vi "Read SMO Address.vi"(8 "error in (no error)":errorcluster, 11 "Instrument in":refnum<class "Instrument.lvclass">) -> (0 "error out":errorcluster, 2 "Address":string, 3 "Instrument out":refnum<class "Instrument.lvclass">)   [LabVIEW 2019, in "Instrument.lvclass"]
uses:
  Instrument.lvclass
  Instrument.lvclass/Instrument.ctl
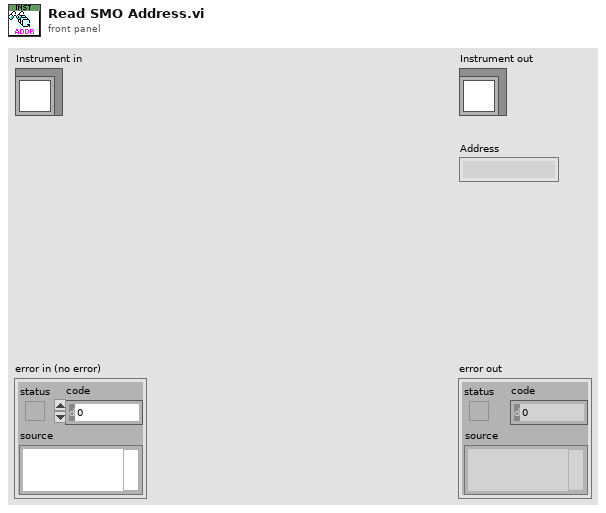
[diagram p1: front panel]
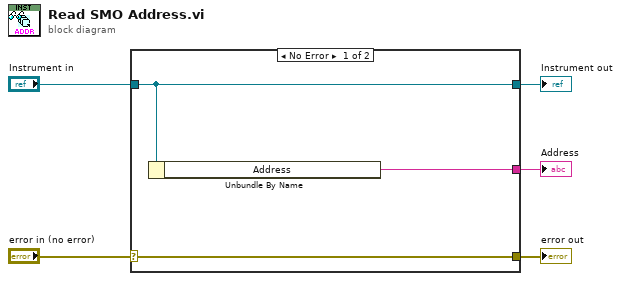
[diagram p0: block diagram]
diagram:
  n1 = case shown="No Error" "error in (no error)" {
    selector: "error in (no error)" -> [w8 w9]
    tunnel: [w8 w9] -> w4
    tunnel: [w6 w10] -> w2
    tunnel: "Instrument in" -> [w6 w10]
    tunnel: [w7 _] -> w1
    frame No Error {
      n2 = Unbundle By Name(w6) -> ("Address"=w7:string)
    }
    frame Error {
    }
  }
  "error out" <- w4
  "Instrument out" <- w2
  "Address" <- w1
